vi "Calculate GRR.vi"(8 "error in (no error)":errorcluster, 10 "Status Monitor":string, 11 "GRR Core in":refnum<class "GRR Core.lvclass">) -> (0 "error out":errorcluster, 2 "Result Data":T1[](array[typedef]), 3 "GRR Core out":refnum<class "GRR Core.lvclass">)   [LabVIEW 2018, in "GRR Core.lvclass"]
uses:
  GRR Core.lvclass
  Result Data Mgr/Typedefs/GRR Result.ctl
  GRR Core.lvclass/GRR Core.ctl
  TestDataMgr/TestDataMgr.lvclass
  Result Data Mgr/Result Data Mgr.lvclass
  Process Bar/Process Bar.lvclass
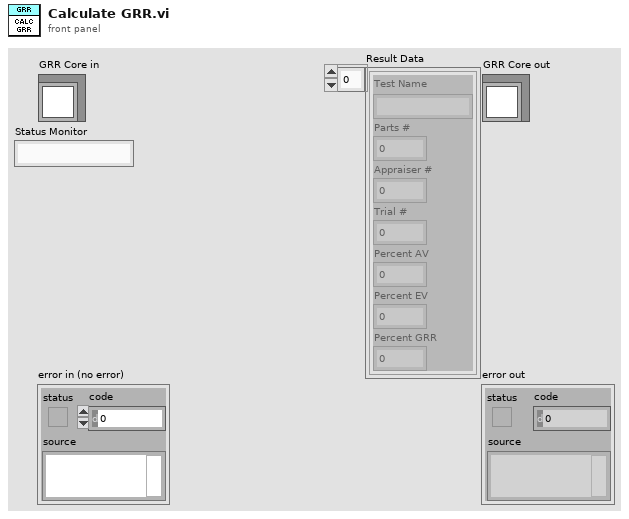
[diagram p1: front panel]
types:
  T1 = typedef "Result Data Mgr.lvclass/GRR Result.ctl" = cluster{"Test Name":string, "Parts #":u8, "Appraiser #":u8, "Trial #":u8, "Percent AV":dbl, "Percent EV":dbl, "Percent GRR":dbl}
  T2 = typedef "Result Data Mgr.lvclass/Session Handle.ctl" = refnum<data-value>
  T3 = typedef "TestDataMgr.lvclass/Session Handle.ctl" = refnum<data-value>
  T4 = typedef "Process Bar.lvclass/Session Handle.ctl" = refnum<data-value>
  T5 = typedef "TestDataMgr.lvclass/Test Data All.ctl" = cluster{"Test Name":string, "Test Limits":T6, "Raw Data Per Tester":T7[]}
  T6 = typedef "TestDataMgr.lvclass/Test Limits.ctl" = cluster{"High":dbl, "Low":dbl}
  T7 = typedef "TestDataMgr.lvclass/Test Raw Data.ctl" = cluster{"Data":dbl[][], "Tester#":u8}
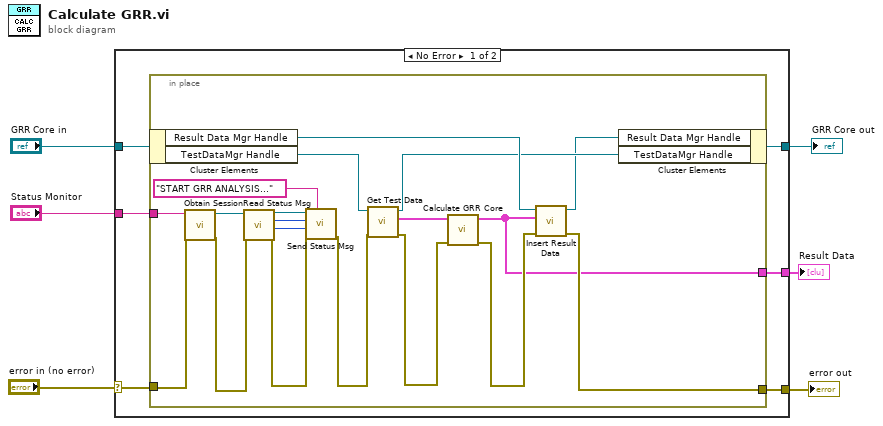
[diagram p0: block diagram]
diagram:
  n1 = case shown="No Error" "error in (no error)" {
    selector: "error in (no error)" -> [w12 w33]
    tunnel: [w9 w33] -> w5
    tunnel: [w10 w32] -> w3
    tunnel: "GRR Core in" -> [w11 w32]
    tunnel: [w8 _] -> w2
    tunnel: "Status Monitor" -> [w7 _]
    frame No Error {
      n2 = in-place {
        in-place-border: w12 -> [w22]
        in-place-border: [w25] -> w9
        in-place-border: [w23] -> w8
        in-place-border: w7 -> [w21]
        n3 = in-place-cluster #1(w11) -> ("Result Data Mgr Handle"=w28:T2, "TestDataMgr Handle"=w27:T3)
        n4 = call "Obtain Session.vi"("error in (no error)"=w22, "Session  Name ()"=w21) -> ("error out"=w17:errorcluster, "Session Handle"=w18:T4)  [unwired: 8 in]
        n5 = call "Read Status Msg.vi"("error in (no error)"=w17, "Session Handle in"=w18) -> ("error out"=w16:errorcluster, "Process Max"=w13:u16, "Process Bar"=w14:u8, "Session Handle out"=w15:T4)  [unwired: 5 in, 1 out]
        n6 = call "Send Status Msg.vi"("Status Msg"="START GRR ANALYSIS...", "error in (no error)"=w16, "Process Max"=w13, "Process Bar"=w14, "Session Handle in"=w15) -> ("error out"=w20:errorcluster)  [unwired: 5 in, 1 out]
        n7 = call "Get Test Data.vi"("error in (no error)"=w20, "Session Handle in"=w27) -> ("error out"=w30:errorcluster, "Test Data"=w31:T5[], "Session Handle out"=w26:T3)  [unwired: 7 in]
        n8 = call "Calculate GRR Core.vi"("error in (no error)"=w30, "Test Data"=w31) -> ("error out"=w29:errorcluster, "Result Data"=w23:T1[])  [unwired: 8 in]
        n9 = call "Insert Result Data.vi"("error in (no error)"=w29, "GRR Results"=w23, "Session Handle in"=w28) -> ("error out"=w25:errorcluster, "Session Handle out"=w24:T2)  [unwired: 7 in]
        n10 = in-place-cluster #1("Result Data Mgr Handle"=w24, "TestDataMgr Handle"=w26) -> (w10:refnum<class "GRR Core.lvclass">)
      }
    }
    frame Error {
    }
  }
  "error out" <- w5
  "GRR Core out" <- w3
  "Result Data" <- w2
